vi "Dashboard Receive Packet.vi"(11 "connection ID":refnum<k16>) -> ()   [LabVIEW 2016]
uses:
  Common Code/Dashboard Control Data.ctl
  Common Code/Drivetrain Settings.ctl
  Common Code/PID Gains.ctl
  Common Code/Input Modifier.ctl
  Common Code/Intake Presets.ctl
  Common Code/Shooter Presets.ctl
  Common Code/Vision Target Packet.ctl
  Common Code/Drivetrain Encoder Values.ctl
  Common Code/Encoder Values.ctl
  Common Code/Auto Agitator Settings.ctl
  Common Code/Climber Settings.ctl
  Common Code/LED Global Data.ctl
  Robot Global Data.vi
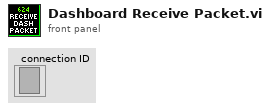
[diagram p1: front panel]
types:
  T1 = typedef "Dashboard Control Data.ctl" = cluster{"Drivetrain Settings":T2, "Intake Presets ":T5, "Shooter Presets":T6, "Vision Target Packet":T7, "Auton Presets":cluster{"Start Position":dbl}, "Drivetrain Encoder Values":T8, "Drivetrain Encoder Settings":cluster{"Left Tick Constant":dbl, "Right Tick Contant":dbl, "Reset Encoders":bool, "Center Tick Constant":dbl}, "Zero Gyro":bool, "Vision Timeout":dbl, "Pressure M":dbl, "Pressure B":dbl, "Auto Agitator":T10, "Climber Settings":T11, "LEDs":T12}
  T2 = typedef "Drivetrain Settings.ctl" = cluster{"Gyro Tolerance":dbl, "Gyro Steer PID Gains":T3, "Y Power Multiplier":dbl, "Turn Power Multiplier":dbl, "Gyro Output":dbl, "Creep Rate":dbl, "Distance Drive PID Gains":T3, "Distance Tolerance":dbl, "Distance Output":dbl, "Strafe Threshold":dbl, "Strafe Correct":bool, "Strafe Tolerance":dbl, "Translate Drive PID Gains":T3, "Strafe Output":dbl, "SC Right":dbl, "SC Left":dbl, "Use Gyro":bool, "Constant Power":bool, "Strafe Power":dbl, "Input Modifier":T4, "SCR Delay":dbl, "SCL Delay":dbl}
  T3 = typedef "PID Gains.ctl" = cluster{"proportional gain (Kc)":dbl, "integral time (Ti, min)":dbl, "derivative time (Td, min)":dbl}
  T4 = typedef "Input Modifier.ctl" = enum16{"None", "Square", "Cube"}
  T5 = typedef "Intake Presets.ctl" = cluster{"Intake Speed ":dbl, "Outake Speed":dbl, "Current Trip Delay":dbl, "Max Current":dbl, "Gear Outtake Motor Delay":dbl, "Gear Intake Motor Delay":dbl, "Gear Intake Pull Up Speed":dbl, "Pusher Delay":dbl, "Release Delay":dbl, "Close Release Delay":dbl}
  T6 = typedef "Shooter Presets.ctl" = cluster{"Key Shot":cluster{"RPM ":dbl, "Hood?":bool}, "Distance Shot":cluster{"RPM":dbl, "Hood?":bool}, "RPM Tolerance":dbl, "Unstuck Delay Time ":dbl, "Initial RPM Increase":dbl, "Warmup Delay":dbl, "Faster Time":dbl, "Shooter PID Gains":cluster{"P":dbl, "I":dbl, "D":dbl, "FF":dbl, "Ramp Rate":dbl, "I Zone":dbl}, "Unstuck Trigger Power":dbl, "Trigger Power":dbl, "Unstuck RPM":dbl, "Agitator Active Power":dbl, "Agitator Idle Power":dbl, "RPM Tuning Range":dbl, "RPM M Tuning Range":dbl}
  T7 = typedef "Vision Target Packet.ctl" = cluster{"Robot Center":dbl, "Center X":dbl, "Center Y":dbl, "Angle":dbl, "Distance":dbl, "Found Target?":bool}
  T8 = typedef "Drivetrain Encoder Values.ctl" = cluster{"Left Encoder":T9, "Center Encoder":T9, "Right Encoder":T9}
  T9 = typedef "Encoder Values.ctl" = cluster{"Distance":dbl, "Speed":dbl, "Tick":dbl}
  T10 = typedef "Auto Agitator Settings.ctl" = cluster{"Enable Auto Agitation":bool, "Continuous Stir":bool, "Continuous Intake":bool, "Alternate In/Outtake":bool, "Wing Delay":dbl, "Stir Delay":dbl, "Intake Delay":dbl, "Wing On Time":dbl, "Wing Off Time":dbl, "Stir On Time":dbl, "Stir Off Time":dbl, "Intake On Time":dbl, "Intake Off Time":dbl, "Stir Power":dbl, "Intake Power":dbl, "Outtake Power":dbl, "Intake Run Time":dbl, "Outtake Run Time":dbl, "Wing$":bool, "Intake":bool, "Stirrer":bool}
  T11 = typedef "Climber Settings.ctl" = cluster{"Climber Power":dbl, "Max Current":dbl, "Avoid Current Trip?":bool}
  T12 = typedef "LED Global Data.ctl" = cluster{"Back":cluster{"Default":string, "Traction":string, "Gear Ready Close":string, "Break On":string, "Gear Loaded":string, "Climb":string, "Gear Ready Far":string, "Unload Gear":string}, "Front":cluster{"Default":string, "Traction":string, "Gear Ready Close":string, "Break On":string, "Gear Loaded":string, "Climb":string, "Gear Ready Far":string, "Unload Gear":string}, "LEDOnTime":dbl, "LEDOffTime":dbl}
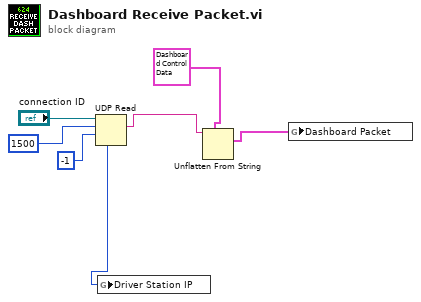
[diagram p0: block diagram]
diagram:
  n1 = UDP Read(connection ID="connection ID", max size (548)=1500, timeout ms (25000)=-1) -> (data out=w3:string, 6:w4:u32)  [unwired: 1 in, 3 out]
  n2 = global write "Robot Global Data.vi" "Driver Station IP"(w4) -> ()
  n3 = Unflatten From String(type=T1 {"Drivetrain Settings"={"Gyro Tolerance"=1.5, "Gyro Steer PID Gains"={"proportional gain (Kc)"=1.0, "integral time (Ti, min)"=0.01, "derivative time (Td, min)"=0.0}, "Y Power Multiplier"=6.0, "Turn Power Multiplier"=5.0, "Gyro Output"=0.85, "Creep Rate"=0.4, "Distance Drive PID Gains"={"proportional gain (Kc)"=1.0, "integral time (Ti, min)"=0.01, "derivative time (Td, min)"=0.0}, "Distance Tolerance"=1.4999999999999998, "Distance Output"=0.85, "Strafe Threshold"=0.4, "Strafe Correct"=FALSE, "Strafe Tolerance"=0.0, "Translate Drive PID Gains"={"proportional gain (Kc)"=1.0, "integral time (Ti, min)"=0.01, "derivative time (Td, min)"=0.0}, "Strafe Output"=0.0, "SC Right"=0.85, "SC Left"=0.85, "Use Gyro"=FALSE, "Constant Power"=FALSE, "Strafe Power"=0.0, "Input Modifier"=enum."None", "SCR Delay"=0.85, "SCL Delay"=0.85}, "Intake Presets "={"Intake Speed "=0.0, "Outake Speed"=0.0, "Current Trip Delay"=0.0, "Max Current"=0.0, "Gear Outtake Motor Delay"=0.0, "Gear Intake Motor Delay"=0.0, "Gear Intake Pull Up Speed"=0.0, "Pusher Delay"=0.0, "Release Delay"=0.0, "Close Release Delay"=0.0}, "Shooter Presets"={"Key Shot"={"RPM "=0.0, "Hood?"=FALSE}, "Distance Shot"={"RPM"=0.0, "Hood?"=FALSE}, "RPM Tolerance"=0.0, "Unstuck Delay Time "=0.0, "Initial RPM Increase"=0.0, "Warmup Delay"=0.0, "Faster Time"=0.0, "Shooter PID Gains"={"P"=0.0, "I"=0.0, "D"=0.0, "FF"=0.0, "Ramp Rate"=0.0, "I Zone"=0.0}, "Unstuck Trigger Power"=0.0, "Trigger Power"=0.0, "Unstuck RPM"=0.0, "Agitator Active Power"=0.0, "Agitator Idle Power"=0.0, "RPM Tuning Range"=0.0, "RPM M Tuning Range"=0.0}, "Vision Target Packet"={"Robot Center"=0.0, "Center X"=0.0, "Center Y"=0.0, "Angle"=0.0, "Distance"=0.0, "Found Target?"=FALSE}, "Auton Presets"={"Start Position"=0.0}, "Drivetrain Encoder Values"={"Left Encoder"={"Distance"=0.0, "Speed"=0.0, "Tick"=0.0}, "Center Encoder"={"Distance"=0.0, "Speed"=0.0, "Tick"=0.0}, "Right Encoder"={"Distance"=0.0, "Speed"=0.0, "Tick"=0.0}}, "Drivetrain Encoder Settings"={"Left Tick Constant"=0.0, "Right Tick Contant"=0.0, "Reset Encoders"=FALSE, "Center Tick Constant"=0.0}, "Zero Gyro"=FALSE, "Vision Timeout"=0.0, "Pressure M"=0.0, "Pressure B"=0.0, "Auto Agitator"={"Enable Auto Agitation"=FALSE, "Continuous Stir"=FALSE, "Continuous Intake"=FALSE, "Alternate In/Outtake"=FALSE, "Wing Delay"=0.0, "Stir Delay"=0.0, "Intake Delay"=0.0, "Wing On Time"=0.0, "Wing Off Time"=0.0, "Stir On Time"=0.0, "Stir Off Time"=0.0, "Intake On Time"=0.0, "Intake Off Time"=0.0, "Stir Power"=0.0, "Intake Power"=0.0, "Outtake Power"=0.0, "Intake Run Time"=0.0, "Outtake Run Time"=0.0, "Wing$"=FALSE, "Intake"=FALSE, "Stirrer"=FALSE}, "Climber Settings"={"Climber Power"=0.0, "Max Current"=0.0, "Avoid Current Trip?"=FALSE}, "LEDs"={"Back"={"Default"="", "Traction"="", "Gear Ready Close"="", "Break On"="", "Gear Loaded"="", "Climb"="", "Gear Ready Far"="", "Unload Gear"=""}, "Front"={"Default"="", "Traction"="", "Gear Ready Close"="", "Break On"="", "Gear Loaded"="", "Climb"="", "Gear Ready Far"="", "Unload Gear"=""}, "LEDOnTime"=0.0, "LEDOffTime"=0.0}} ("Dashboard Packet"), binary string=w3) -> (value=w1:T1)  [unwired: 3 in, 2 out]
  n4 = global write "Robot Global Data.vi" "Dashboard Packet"(w1) -> ()
